vi "Migrate Dependencies.vi"() -> ()   [LabVIEW 2021]
uses:
  measurement_migration_tool/_Measurement Migrator/Migrator/Queue Driver/controls/Queue Operations.ctl
  controls/Data Holder.ctl
  measurement_migration_tool/_Measurement Migrator/Migrator/Queue Driver/Queue Driver.lvlib
panel:
  in  "Plug-in names":string[](array[string])
  in  "Measurement paths":path[](array[path])
  in  "Info":string="Migration done!!"
  in  "Start":bool
  in  "Project path":path=path "C:/Workspace/measurement-migration-tool/src/Test Folder/Shared Test/Shared Test.lvproj"
  # "Dependencies Migration"
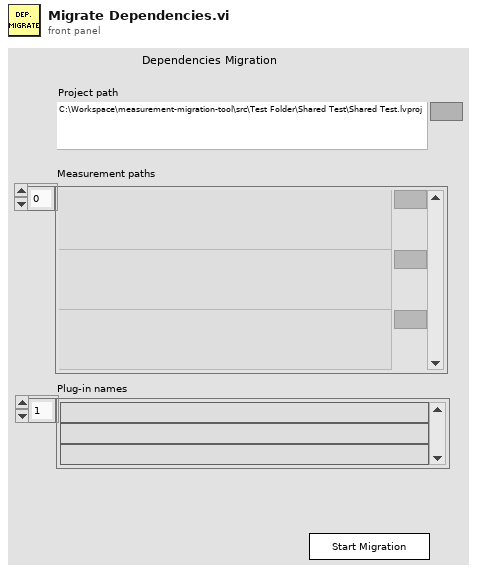
[diagram p1: front panel]
types:
  T1 = typedef "Queue Driver.lvlib/Queue Operations.ctl" = enum16{"Create Q", "Enqueue", "Enqueue N", "Dequeue", "Flush", "Release"}
  T2 = typedef "Data Holder.ctl" = cluster{"Project path":path, "Measurement paths":path[], "Plug-in names":string[]}
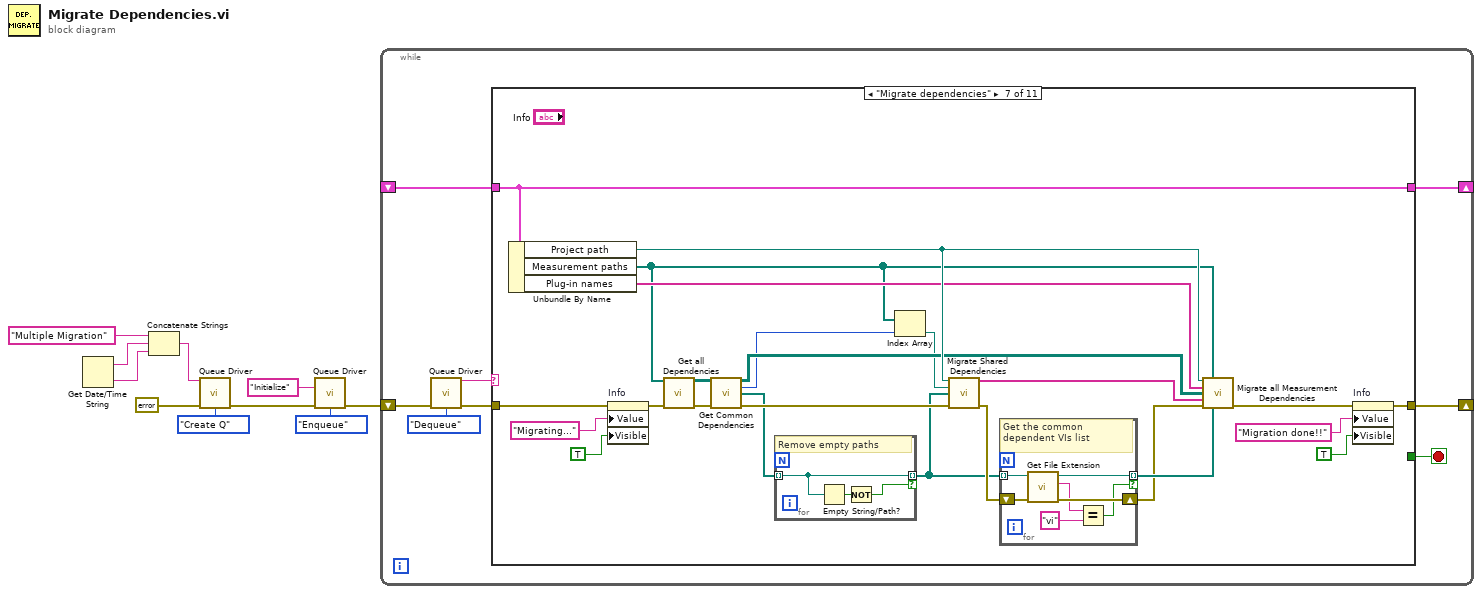
[diagram p0: block diagram]
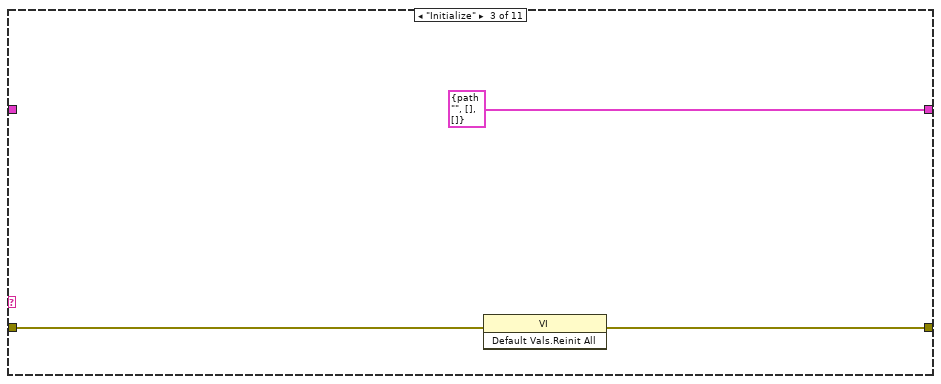
[diagram p4: hidden frame]
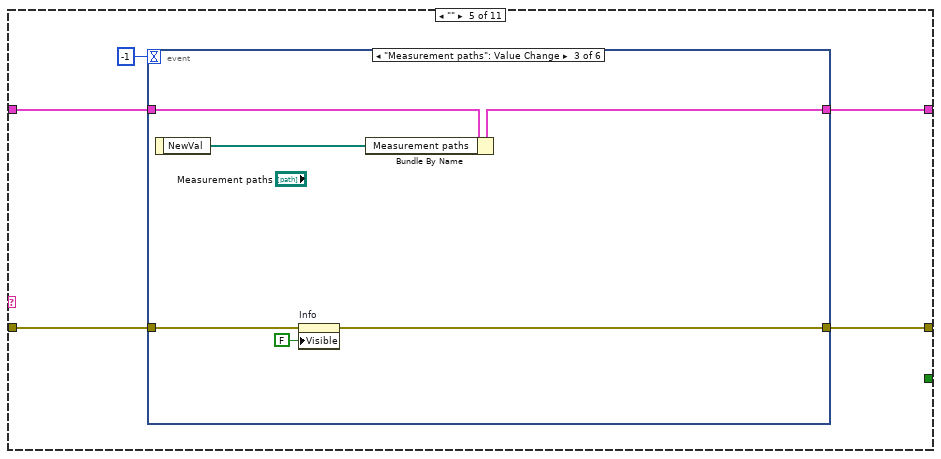
[diagram p6: hidden frame]
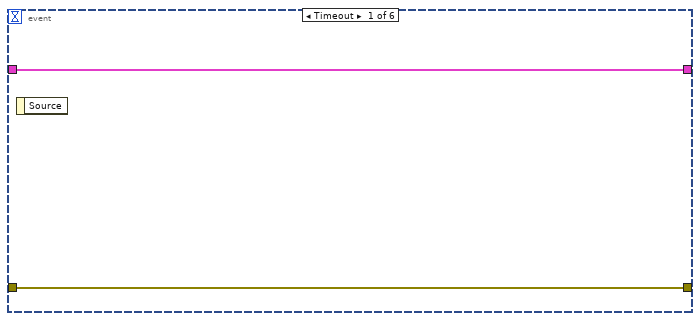
[diagram p7: hidden frame]
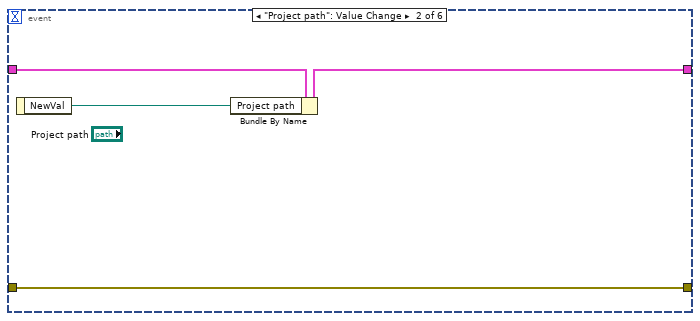
[diagram p8: hidden frame]
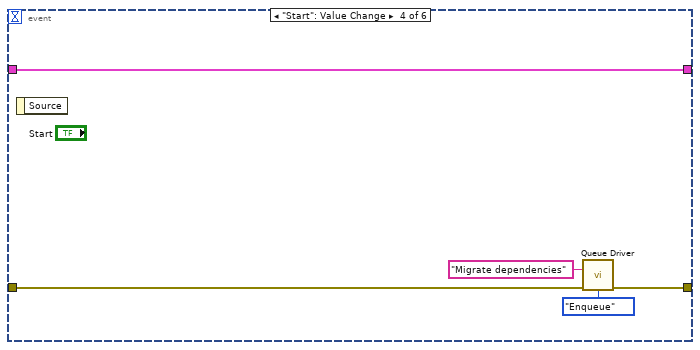
[diagram p9: hidden frame]
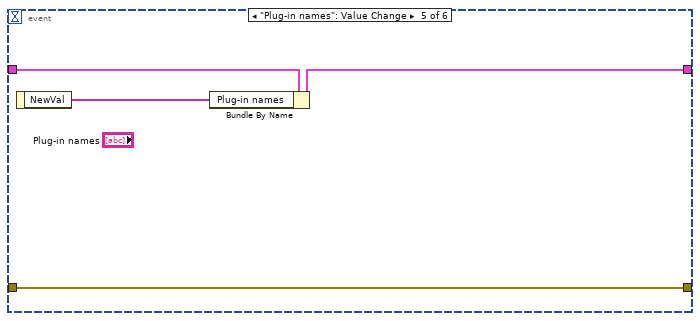
[diagram p10: hidden frame]
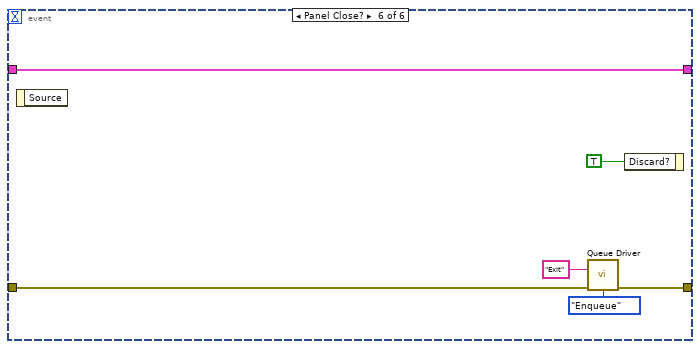
[diagram p11: hidden frame]
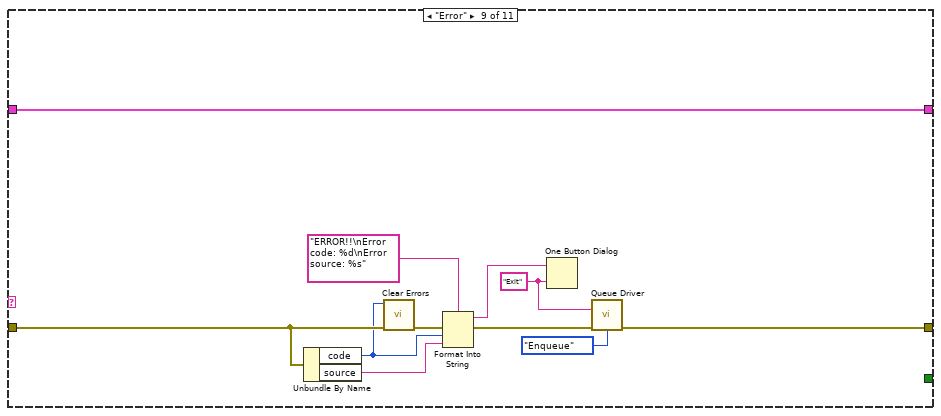
[diagram p14: hidden frame]
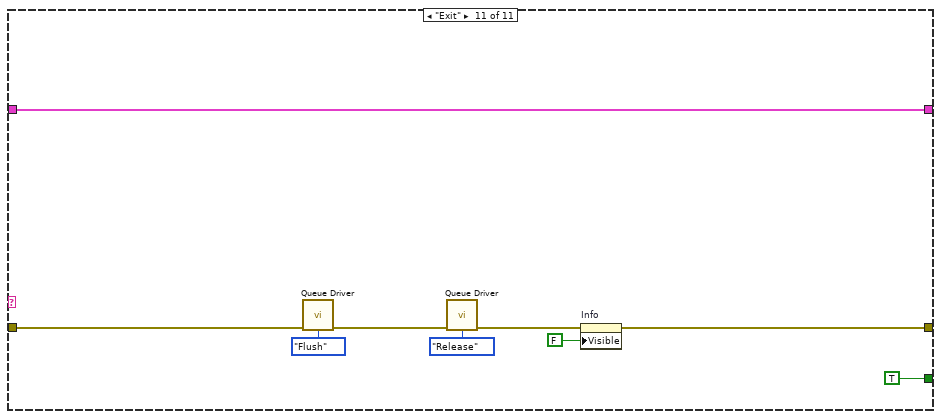
[diagram p16: hidden frame]
diagram:
  n1 = Get Date/Time String() -> (date string=w8:string, time string=w7:string)  [unwired: 3 in]
  n2 = Concatenate Strings("Multiple Migration" ("string"), w8, w7) -> (w5:string)
  n3 = call "Queue Driver.vi"("Name"=w5, "error in (no error)"=errorcluster {"status"=FALSE, "code"=0, "source"=""} ("error constant"), "Q Operations"=Queue_Operations."Create Q") -> ("error out"=w4:errorcluster)  [unwired: 11 in, 1 out]
  n4 = call "Queue Driver.vi"("State"="Initialize", "error in (no error)"=w4, "Q Operations"=Queue_Operations."Enqueue") -> ("error out"=w1:errorcluster)  [unwired: 11 in, 1 out]
  n5 = while {
    shift-right: [w14] -> _
    shift-left: w1 -> [w18]
    shift-right: [w12] -> _
    shift-left: _ -> [w11]
    stop <- w13 stop-if-true
    n6 = call "Queue Driver.vi"("error in (no error)"=w18, "Q Operations"=Queue_Operations."Dequeue") -> ("Dequeued State"=w15:string, "error out"=w17:errorcluster)  [unwired: 12 in]
    n7 = case shown="\"Migrate dependencies\"" w15 {
      tunnel: w17 -> [w20 w22 w25 w27 w32 w61 w62 w97 w107 w110 w119]
      tunnel: [w20 w22 w23 w27 w31 w61 w84 w97 w102 w110 w113] -> w14
      tunnel: [_ _ _ _ _ _ _ _ _ _ TRUE] -> w13
      tunnel: [w19 w21 T2 {"Project path"=path "", "Measurement paths"=[], "Plug-in names"=[]} w26 w28 w60 w85 w96 w99 w109 w114] -> w12
      tunnel: w11 -> [w19 w21 _ w26 w29 w60 w85 w96 w99 w109 w114]
      frame Default {
      }
      frame "**********Initialize**********" {
      }
      frame "Initialize" {
        n8 = invoke class="VI" method="Default Vals.Reinit All"(error in=w25) -> (error out=w23:errorcluster)  [unwired: 2 in, 2 out]
      }
      frame "**********FP related**********" {
      }
      frame "" {
        n9 = event shown="[2] \"Measurement paths\": Value Change" {
          selector: _ -> [_ _ _ _ _ _]
          dyn-events: _ -> [_ _ _ _ _ _]
          timeout: -1 -> [_ _ _ _ _ _]
          tunnel: w32 -> [w34 w38 w42 w49 w53 w58]
          tunnel: [w34 w38 w41 w48 w53 w57] -> w31
          tunnel: w29 -> [w33 w37 w44 w45 w52 w54]
          tunnel: [w33 w36 w43 w45 w51 w54] -> w28
          event Timeout {
            n10 = event-data() -> ()  [unwired: 1 in, 1 out]
          }
          event "Project path": Value Change {
            n11 = event-data() -> ("NewVal"=w35:path)  [unwired: 1 in]
            n12 = Bundle By Name(cluster=w37, "Project path"=w35) -> (w36:T2)
          }
          event "Measurement paths": Value Change {
            n13 = event-data() -> ("NewVal"=w39:path[])  [unwired: 1 in]
            n14 = property on="Info" class="Str"(error in=w42, "Visible"=FALSE) -> (error out=w41:errorcluster)  [unwired: 1 in, 1 out]
            n15 = Bundle By Name(cluster=w44, "Measurement paths"=w39) -> (w43:T2)
          }
          event "Start": Value Change {
            n16 = event-data() -> ()  [unwired: 1 in, 1 out]
            n17 = call "Queue Driver.vi"("State"="Migrate dependencies", "error in (no error)"=w49, "Q Operations"=Queue_Operations."Enqueue") -> ("error out"=w48:errorcluster)  [unwired: 11 in, 1 out]
          }
          event "Plug-in names": Value Change {
            n18 = event-data() -> ("NewVal"=w50:string[])  [unwired: 1 in]
            n19 = Bundle By Name(cluster=w52, "Plug-in names"=w50) -> (w51:T2)
          }
          event Panel Close? {
            n20 = event-data() -> ()  [unwired: 1 in, 1 out]
            n21 = call "Queue Driver.vi"("State"="Exit", "error in (no error)"=w58, "Q Operations"=Queue_Operations."Enqueue") -> ("error out"=w57:errorcluster)  [unwired: 11 in, 1 out]
            n22 = event-data("Discard?"=TRUE) -> ()  [unwired: 1 in, 1 out]
          }
        }
      }
      frame "**********Functionality**********" {
      }
      frame "Migrate dependencies" {
        n23 = Unbundle By Name(w85) -> ("Project path"=w77:path, "Measurement paths"=w70:path[], "Plug-in names"=w75:string[])
        n24 = property on="Info" class="Str"(error in=w62, "Value"="Migrating..." ("Info"), "Visible"=TRUE) -> (error out=w65:errorcluster)  [unwired: 1 in, 1 out]
        n25 = call "Get all Dependencies.vi"("Measurement paths"=w70, "error in (no error)"=w65) -> ("All dependencies"=w79:path[][], "error out"=w81:errorcluster)  [unwired: 11 in, 1 out]
        n26 = call "Get Common Dependencies.vi"("All dependencies"=w79, "error in (no error)"=w81) -> ("Measurement dependencies"=w76:path[][], "Measurement index"=w67:i32, "Common dependencies"=w68:path[], "error out"=w80:errorcluster)  [unwired: 10 in]
        n27 = for {
          tunnel: [w86] -> w66 mode=indexing if=w87
          tunnel: w68 -> [w86] mode=indexing
          # "Remove empty paths"
          n28 = Empty String/Path?(string/path=w86) -> (empty?=w88:bool)
          n29 = Not(x=w88) -> (.not. x?=w87:bool)
        }
        n30 = Index Array(array=w70, index=w67) -> (element=w69:path)
        n31 = call "Migrate Shared Dependencies.vi"("Project path"=w77, "Measurement path"=w69, "Common dependencies"=w66, "error in (no error)"=w80) -> ("Outside items"=w74:string[], "error out"=w72:errorcluster)  [unwired: 10 in]
        n32 = for {
          shift-right: [w94] -> w71
          shift-left: w72 -> [w95]
          tunnel: [w90] -> w73 mode=indexing if=w91
          tunnel: w66 -> [w89] mode=indexing
          # "Get the common dependent VIs list"
          n33 = call <vilib>:"Get File Extension.vi"("error in (no error)"=w95, "file"=w89) -> ("error out"=w94:errorcluster, "lowercase file extension"=w92:string, "dup file"=w90:path)  [unwired: 5 in, 2 out]
          n34 = Equal?(x=w92, y="vi" ("x")) -> (x = y?=w91:bool)
        }
        n35 = call "Migrate all Measurement Dependencies.vi"("Project path"=w77, "Measurement paths"=w70, "Plug-in names"=w75, "Measurement dependencies"=w76, "Outside items"=w74, "error in (no error)"=w71, "Shared dependent VIs"=w73) -> ("error out"=w78:errorcluster)  [unwired: 8 in]
        n36 = property on="Info" class="Str"(error in=w78, "Value"="Migration done!!" ("Info"), "Visible"=TRUE) -> (error out=w84:errorcluster)  [unwired: 1 in, 1 out]
      }
      frame "**********Error**********" {
      }
      frame "Error" {
        w100 = "Exit" ("button name (\"OK\")")
        n37 = Unbundle By Name(w107) -> ("code"=w98:i32, "source"=w106:string)
        n38 = call <vilib>:"Clear Errors.vi"("error in (no error)"=w107, "specific error code to clear (0: all)"=w98) -> ("error out"=w108:errorcluster)  [unwired: 4 in, 1 out]
        n39 = Format Into String(format string="ERROR!!\nError code: %d\nError source: %s", error in=w108, w98, w106) -> (resulting string=w104:string, error out=w103:errorcluster)  [unwired: 1 in]
        n40 = One Button Dialog(message=w104, button name ("OK")=w100) -> ()  [unwired: 1 out]
        n41 = call "Queue Driver.vi"("State"=w100, "error in (no error)"=w103, "Q Operations"=Queue_Operations."Enqueue") -> ("error out"=w102:errorcluster)  [unwired: 11 in, 1 out]
      }
      frame "**********Exit**********" {
      }
      frame "Exit" {
        n42 = call "Queue Driver.vi"("error in (no error)"=w119, "Q Operations"=Queue_Operations."Flush") -> ("error out"=w118:errorcluster)  [unwired: 12 in, 1 out]
        n43 = call "Queue Driver.vi"("error in (no error)"=w118, "Q Operations"=Queue_Operations."Release") -> ("error out"=w112:errorcluster)  [unwired: 12 in, 1 out]
        n44 = property on="Info" class="Str"(error in=w112, "Visible"=FALSE) -> (error out=w113:errorcluster)  [unwired: 1 in, 1 out]
      }
    }
  }
